vi "ingest.trigger_file_ingest-new_dataset.vi"(5 "prefixTreeDelimiter":string, 6 "Properties and Labels":T1, 7 "ISO8601 Timestamp Series Name":string, 8 "error in":errorcluster, 9 "Title and Description":cluster{"Title":string, "Description":string}, 10 "S3 Path to File":string, 11 "Nominal Client in":refnum<class "Nominal Client.lvclass">) -> (0 "error out":errorcluster, 1 "JSON out":string, 2 "Information":T2, 3 "Nominal Client out":refnum<class "Nominal Client.lvclass">, 4 "Response":string)   [LabVIEW 2020, in "Nominal Client.lvclass"]
doc: "Triggers an ingest job of a new file, allowing either creating a new dataset or uploading to an existing one."
uses:
  Nominal Client.lvclass
  ae647589-d40a-40ab-8bd3-12ed03615a29.vi
  49ecdc87-d06e-40b5-807d-cfeea5b09dd4.vi
  4b965f09-dc68-4d5e-a5c1-32d476accfd4.vi
  <vilib>/JDP Science/JSONtext/Variant to JSON Text.vi
  <vilib>/JDP Science/JSONtext/Array of Variants to JSON Object.vi
  <vilib>/JDP Science/JSONtext/Set Item.vi
  <vilib>/JDP Science/JSONtext/JSON text to Variant.vi
  <vilib>/JDP Science/JSONtext/LVClass Serializer/JSONtext LVClass Serializer.lvclass
  Nominal Client.lvclass/Nominal Client.ctl
  <vilib>/JDP Science/JSONtext/JSONtext.lvlib
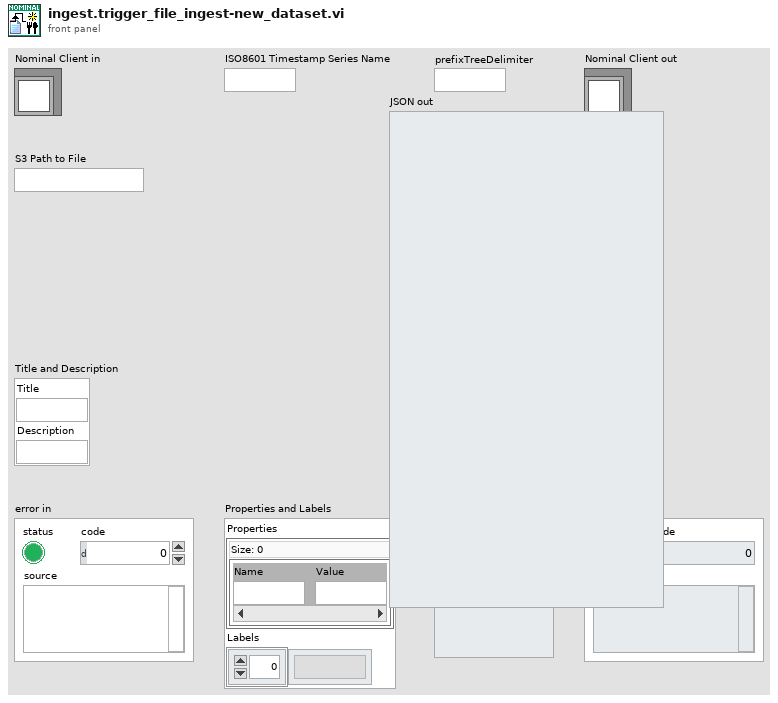
[diagram p1: front panel]
types:
  T1 = cluster{"Properties":map{string, string}, "Labels":string[]}
  T2 = cluster{"datasetRid":string, "datasetFileId":string, "asyncHandle":cluster{"rid":string}}
  T3 = cluster{"type":string, "s3":cluster{"path":string}}
  T4 = cluster{"timestamp_metadata":cluster{"series_name":string, "timestamp_type":string}}
  T5 = cluster{"type":string, "newDataset":cluster{"properties":string, "labels":string[], "datasetName":string, "datasetDescription":string, "channelConfig":cluster{"prefixTreeDelimiter":string}}}
  T6 = cluster{"source":cluster{"type":string, "s3":cluster{"path":string}}, "destination":cluster{"type":string, "newDataset":cluster{"properties":string, "labels":string[], "datasetName":string, "datasetDescription":string, "channelConfig":cluster{"prefixTreeDelimiter":string}}}, "source_metadata":cluster{"timestamp_metadata":cluster{"series_name":string, "timestamp_type":string}}}
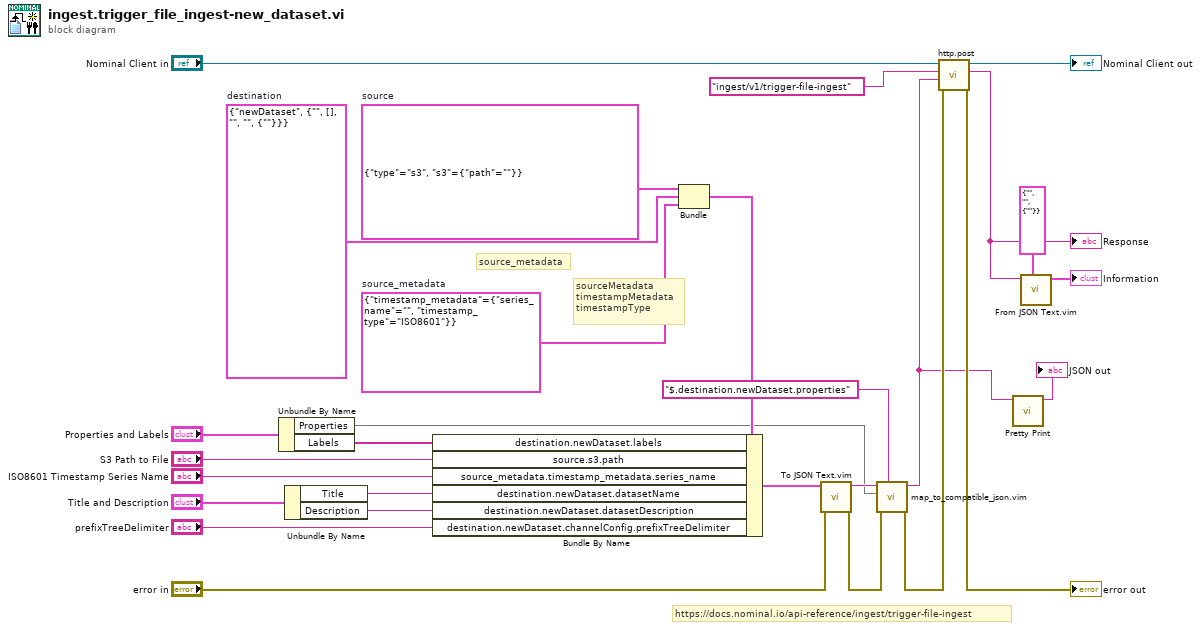
[diagram p0: block diagram]
diagram:
  w23 = T3 {"type"="s3", "s3"={"path"=""}}  # source
  w24 = T4 {"timestamp_metadata"={"series_name"="", "timestamp_type"="ISO8601"}}  # source_metadata
  w25 = T5 {"type"="newDataset", "newDataset"={"properties"="", "labels"=[], "datasetName"="", "datasetDescription"="", "channelConfig"={"prefixTreeDelimiter"=""}}}  # destination
  # "sourceMetadata\ntimestampMetadata\ntimestampType"
  # "source_metadata"
  # "https://docs.nominal.io/api-reference/ingest/trigger-file-ingest"
  n1 = Unbundle By Name("Properties and Labels") -> ("Properties"=w8:map{string, string}, "Labels"=w9:string[])
  n2 = Unbundle By Name("Title and Description") -> ("Title"=w5:string, "Description"=w6:string)
  n3 = Bundle("source"=w23, "destination"=w25, "source_metadata"=w24) -> (w22:T6)  [unwired: 1 in]
  n4 = Bundle By Name(cluster=w22, "destination.newDataset.labels"=w9, "source.s3.path"="S3 Path to File", "source_metadata.timestamp_metadata.series_name"="ISO8601 Timestamp Series Name", "destination.newDataset.datasetName"=w5, "destination.newDataset.datasetDescription"=w6, "destination.newDataset.channelConfig.prefixTreeDelimiter"="prefixTreeDelimiter") -> (w21:T6)
  n5 = call "To JSON Text.vim"("error in (no error)"="error in", "Anything"=w21) -> ("error out"=w11:errorcluster, "<JSON>"=w13:string)  [unwired: 8 in]
  n6 = call "map_to_compatible_json.vim"("JSON Path"="$.destination.newDataset.properties" ("Data Name"), "error in"=w11, "Map"=w8, "JSON in"=w13) -> ("error out"=w12:errorcluster, "JSON out"=w4:string)  [unwired: 6 in]
  n7 = call "http.post.vi"("error in"=w12, "Request body"=w4, "Path"="ingest/v1/trigger-file-ingest", "Nominal Client in"="Nominal Client in") -> ("error out"=→"error out":errorcluster, "Response"=w16:string, "Nominal Client out"=→"Nominal Client out":refnum<class "Nominal Client.lvclass">)  [unwired: 4 in, 1 out]
  "Response" <- w16
  n8 = call <vilib>:"Pretty Print.vi"("JSON"=w4) -> ("<JSON>"=→"JSON out":string)  [unwired: 8 in, 2 out]
  n9 = call "From JSON Text.vim"("Data Type and Default Value"=T2 {"datasetRid"="", "datasetFileId"="", "asyncHandle"={"rid"=""}} ("Information"), "JSON"=w16) -> ("Data out"=→"Information":T2)  [unwired: 8 in, 1 out]
